vi "GT Get Card No.vi"(8 "error in (no error)":errorcluster caption="错误输入（无错误）", 11 "pIndex":i16) -> (0 "error out":errorcluster caption="错误输出", 2 "function return":i16, 3 "pIndex out":i16)   [LabVIEW 2014, in "gts.lvlib"]
doc: "GT_API GT_GetCardNo(short *pIndex);"
uses:
  gts.lvlib
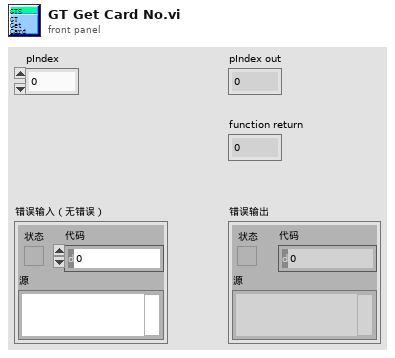
[diagram p1: front panel]
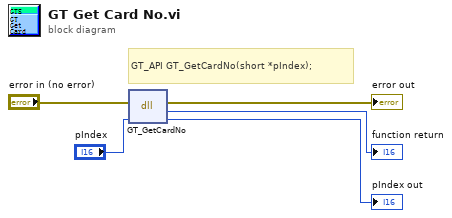
[diagram p0: block diagram]
diagram:
  # "GT_API GT_GetCardNo(short *pIndex);"
  n1 = dll-call lib="PTH2habs D固高科技资料GTS控制卡GTS卡18年上半年资料dllVC32bit\nmulti_cardgts.*" fn="GT_GetCardNo"(error in="error in (no error)", "pIndex"="pIndex") -> (error out=→"error out":errorcluster, →"function return":i16, "pIndex"=→"pIndex out":i16)  [unwired: 2 in, 1 out]
